vi "Data_Base_logging.vi"() -> (1 "Logging On?":bool, 2 "Close Loop with Pitot?":bool, 3 "Rig Name":string="Run EnFlo Hub.vi", 4 "DB Setup files":string[](array[string])=["EnFlo Tun DB setup.xls", "A Tunnel DB setup.xls", "D Tunnel DB setup.xls", "Aero Tunnel DB setup.xls"] caption="DB Setup files (from EnFlo Tun Setup Global)")   [LabVIEW 2012]
uses:
  Controls/Server_Comms.ctl
  Globals/Preference_global.vi
  ADAM Server/Sub VI's/Exp conditions/EnFlo_Tun_Setup_global.vi
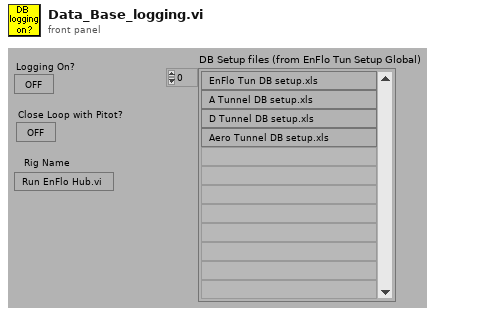
[diagram p1: front panel]
types:
  T1 = typedef "Server_Comms.ctl" = enum16{"Server Link Healthy", "Do Not Link To Server"}
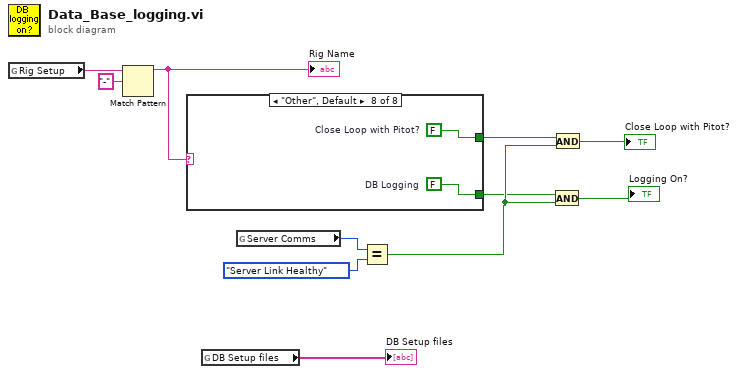
[diagram p0: block diagram]
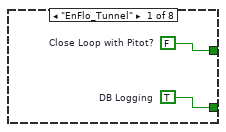
[diagram p2: hidden frame]
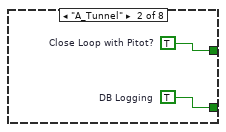
[diagram p3: hidden frame]
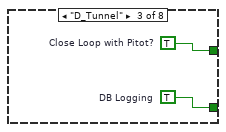
[diagram p4: hidden frame]
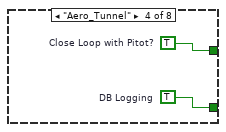
[diagram p5: hidden frame]
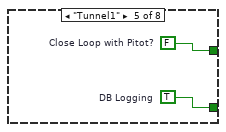
[diagram p6: hidden frame]
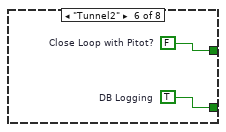
[diagram p7: hidden frame]
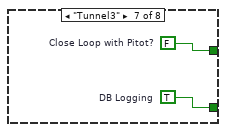
[diagram p8: hidden frame]
diagram:
  n1 = global read "Preference_global.vi" "Rig Setup"() -> (w4:string)
  n2 = Match Pattern(string=w4, regular expression="-") -> (before substring=w2:string)  [unwired: 4 out]
  "Rig Name" <- w2
  n3 = case shown="\"Other\", Default" w2 {
    tunnel: [w13 w15 w17 w19 w21 w23 w25 w27] -> w6
    tunnel: [w12 w14 w16 w18 w20 w22 w24 w26] -> w5
    frame "EnFlo_Tunnel" {
      w12 = TRUE  # DB Logging
      w13 = FALSE  # Close Loop with Pitot?
    }
    frame "A_Tunnel" {
      w14 = TRUE  # DB Logging
      w15 = TRUE  # Close Loop with Pitot?
    }
    frame "D_Tunnel" {
      w16 = TRUE  # DB Logging
      w17 = TRUE  # Close Loop with Pitot?
    }
    frame "Aero_Tunnel" {
      w18 = TRUE  # DB Logging
      w19 = TRUE  # Close Loop with Pitot?
    }
    frame "Tunnel1" {
      w20 = TRUE  # DB Logging
      w21 = FALSE  # Close Loop with Pitot?
    }
    frame "Tunnel2" {
      w22 = TRUE  # DB Logging
      w23 = FALSE  # Close Loop with Pitot?
    }
    frame "Tunnel3" {
      w24 = TRUE  # DB Logging
      w25 = FALSE  # Close Loop with Pitot?
    }
    frame "Other", Default {
      w26 = FALSE  # DB Logging
      w27 = FALSE  # Close Loop with Pitot?
    }
  }
  n4 = global read "EnFlo_Tun_Setup_global.vi" "DB Setup files"() -> (→"DB Setup files":string[])
  n5 = global read "Preference_global.vi" "Server Comms"() -> (w10:T1)
  n6 = Equal?(x=w10, y=Server_Comms."Server Link Healthy" ("Server Comms")) -> (x = y?=w7:bool)
  n7 = And(x=w5, y=w7) -> (x .and. y?=→"Logging On?":bool)
  n8 = And(x=w6, y=w7) -> (x .and. y?=→"Close Loop with Pitot?":bool)
